vi "WAV_Even.vi"(11 "string in":string) -> (3 "string out":string)   [LabVIEW 2022 SP3]
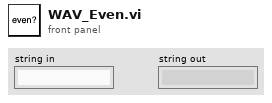
[diagram p1: front panel]
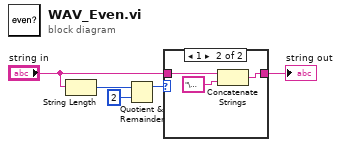
[diagram p0: block diagram]
diagram:
  n1 = String Length(string="string in") -> (length=w5:i32)
  n2 = Quotient & Remainder(x=w5, y=2) -> (x-y*floor(x/y)=w3:i32)  [unwired: 1 out]
  n3 = case shown="1" w3 {
    tunnel: [w6 w8] -> w2
    tunnel: "string in" -> [w6 w9]
    frame 0, Default {
    }
    frame 1 {
      n4 = Concatenate Strings(w9, "\u0000" ("string")) -> (w8:string)
    }
  }
  "string out" <- w2
